vi "FlatToRichnixnet_grpc_GetPropertyResponse.vi"(5 "OutputClusterType":T1, 11 "InputCluster":T2) -> (3 "OutputCluster":T1)   [LabVIEW 2025, in "grpc-xnet_client.lvlib"]
uses:
  grpc-xnet_client.lvlib
  nixnet_grpc_GetPropertyResponse_Flat.ctl
  nixnet_grpc_U32Array_Flat.ctl
  nidevice_grpc_Session_Flat.ctl
  nixnet_grpc_DbRefArray_Flat.ctl
  nixnet_grpc_DeviceRefArray_Flat.ctl
  nixnet_grpc_InterfaceRefArray_Flat.ctl
  nixnet_grpc_EptRxFilterArray_Flat.ctl
  nixnet_grpc_EptRxFilter_Flat.ctl
  nixnet_grpc_GetPropertyResponse.ctl
  nixnet_grpc_GetPropertyResponse_property_value/nixnet_grpc_GetPropertyResponse_property_value.lvclass
  nixnet_grpc_GetPropertyResponse_property_value/nixnet_grpc_GetPropertyResponse_property_value.lvclass/nixnet_grpc_GetPropertyResponse_property_value.ctl
  FlatToRichnixnet_grpc_EptRxFilter.vi
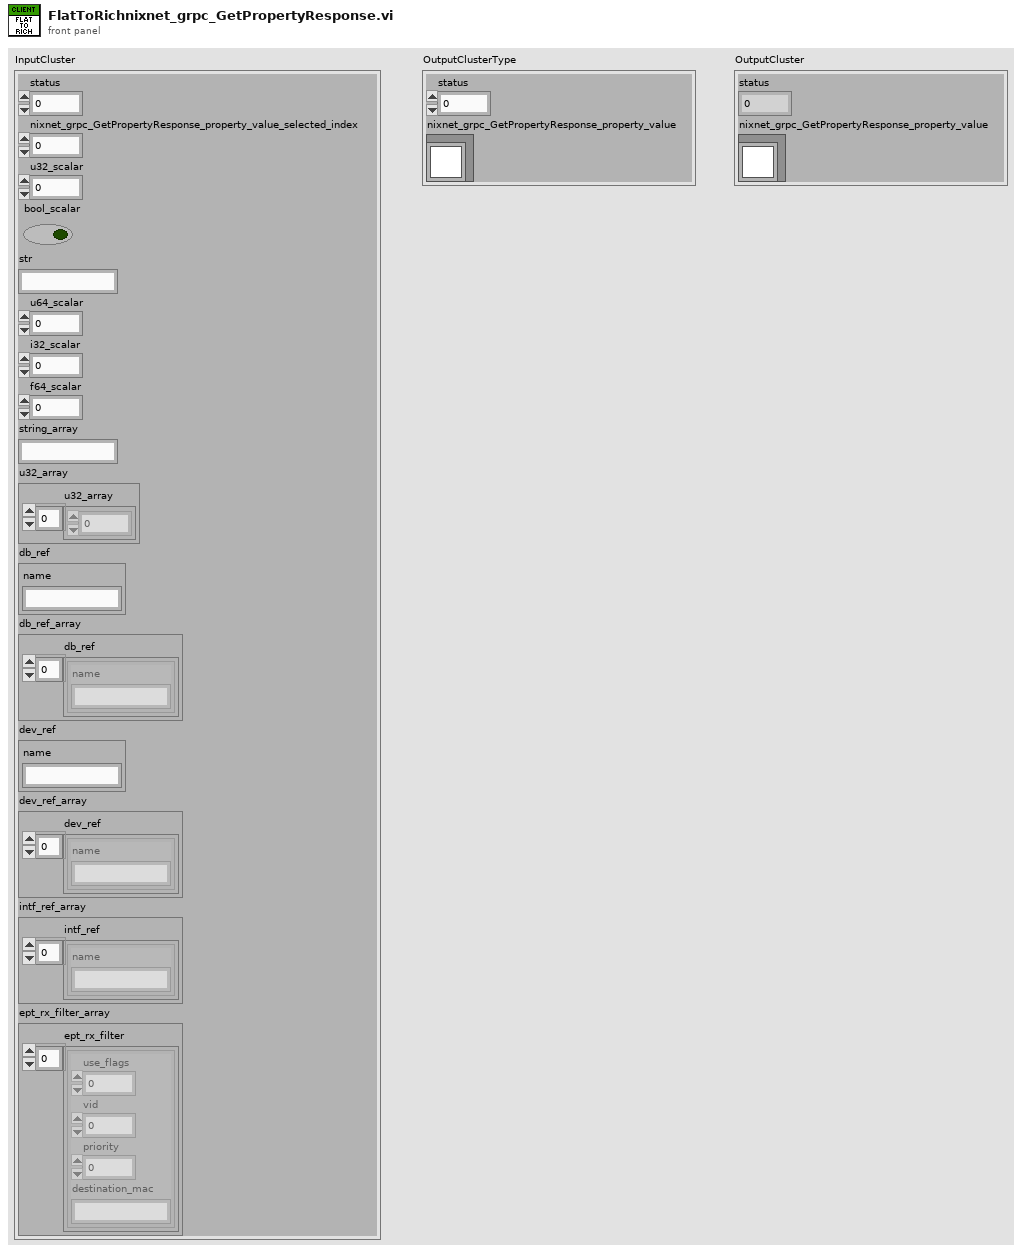
[diagram p1: front panel]
types:
  T1 = typedef "grpc-xnet_client.lvlib/nixnet_grpc_GetPropertyResponse.ctl" = cluster{"status":i32, "nixnet_grpc_GetPropertyResponse_property_value":refnum<class "nixnet_grpc_GetPropertyResponse_property_value.lvclass">}
  T2 = typedef "grpc-xnet_client.lvlib/nixnet_grpc_GetPropertyResponse_Flat.ctl" = cluster{"status":i32, "nixnet_grpc_GetPropertyResponse_property_value_selected_index":i32, "u32_scalar":u32, "bool_scalar":bool, "str":string, "u64_scalar":u64, "i32_scalar":i32, "f64_scalar":dbl, "string_array":string, "u32_array":T3, "db_ref":T4, "db_ref_array":T5, "dev_ref":T4, "dev_ref_array":T6, "intf_ref_array":T7, "ept_rx_filter_array":T8}
  T3 = typedef "grpc-xnet_client.lvlib/nixnet_grpc_U32Array_Flat.ctl" = cluster{"u32_array":u32[]}
  T4 = typedef "grpc-xnet_client.lvlib/nidevice_grpc_Session_Flat.ctl" = cluster{"name":string}
  T5 = typedef "grpc-xnet_client.lvlib/nixnet_grpc_DbRefArray_Flat.ctl" = cluster{"db_ref":T4[]}
  T6 = typedef "grpc-xnet_client.lvlib/nixnet_grpc_DeviceRefArray_Flat.ctl" = cluster{"dev_ref":T4[]}
  T7 = typedef "grpc-xnet_client.lvlib/nixnet_grpc_InterfaceRefArray_Flat.ctl" = cluster{"intf_ref":T4[]}
  T8 = typedef "grpc-xnet_client.lvlib/nixnet_grpc_EptRxFilterArray_Flat.ctl" = cluster{"ept_rx_filter":T9[]}
  T9 = typedef "grpc-xnet_client.lvlib/nixnet_grpc_EptRxFilter_Flat.ctl" = cluster{"use_flags":u32, "vid":u32, "priority":u32, "destination_mac":string}
  T10 = typedef "grpc-xnet_client.lvlib/nixnet_grpc_U32Array.ctl" = cluster{"u32_array":u32[]}
  T11 = typedef "grpc-xnet_client.lvlib/nidevice_grpc_Session.ctl" = cluster{"name":string}
  T12 = typedef "grpc-xnet_client.lvlib/nixnet_grpc_DbRefArray.ctl" = cluster{"db_ref":T11[]}
  T13 = typedef "grpc-xnet_client.lvlib/nixnet_grpc_DeviceRefArray.ctl" = cluster{"dev_ref":T11[]}
  T14 = typedef "grpc-xnet_client.lvlib/nixnet_grpc_InterfaceRefArray.ctl" = cluster{"intf_ref":T11[]}
  T15 = typedef "grpc-xnet_client.lvlib/nixnet_grpc_EptRxFilterArray.ctl" = cluster{"ept_rx_filter":T16[]}
  T16 = typedef "grpc-xnet_client.lvlib/nixnet_grpc_EptRxFilter.ctl" = cluster{"use_flags":u32, "vid":u32, "priority":u32, "destination_mac":string}
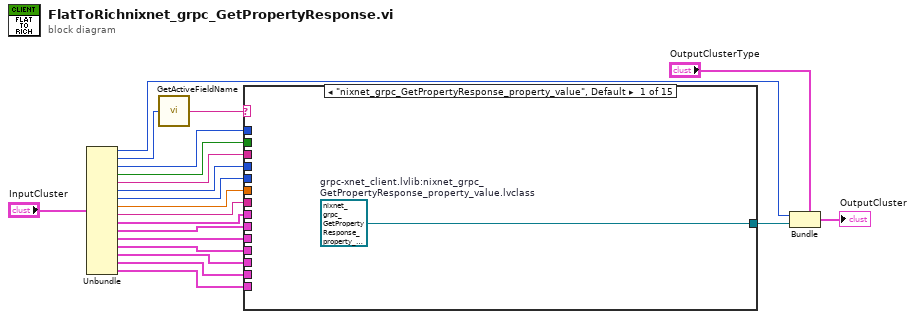
[diagram p0: block diagram]
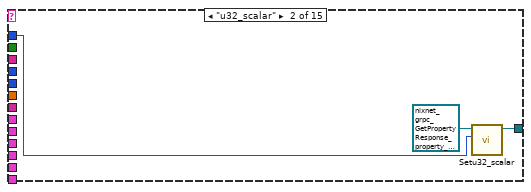
[diagram p2: hidden frame]
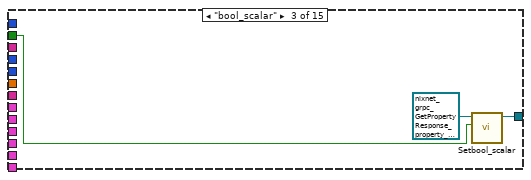
[diagram p3: hidden frame]
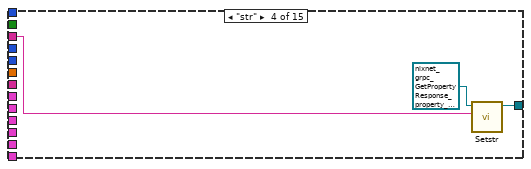
[diagram p4: hidden frame]
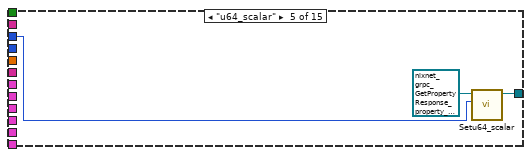
[diagram p5: hidden frame]
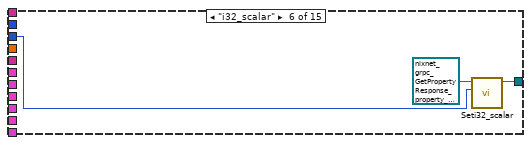
[diagram p6: hidden frame]
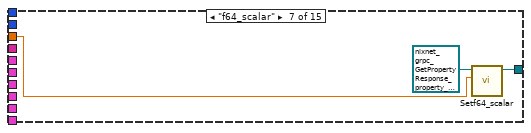
[diagram p7: hidden frame]
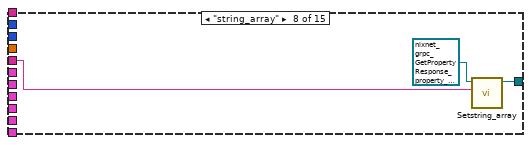
[diagram p8: hidden frame]
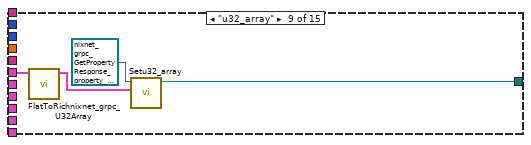
[diagram p9: hidden frame]
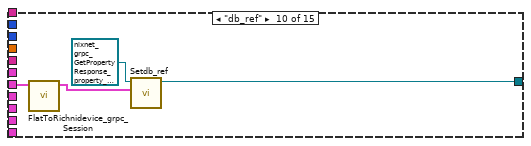
[diagram p10: hidden frame]
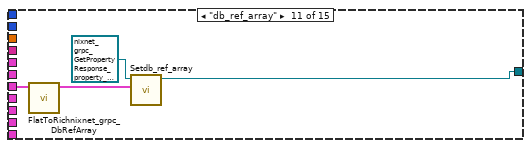
[diagram p11: hidden frame]
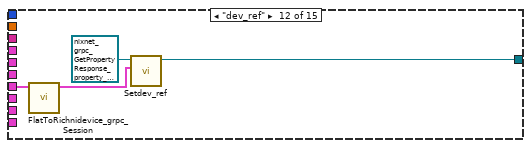
[diagram p12: hidden frame]
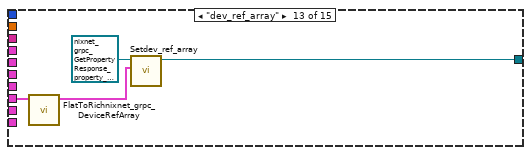
[diagram p13: hidden frame]
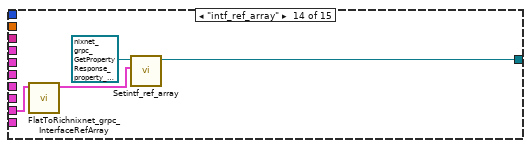
[diagram p14: hidden frame]
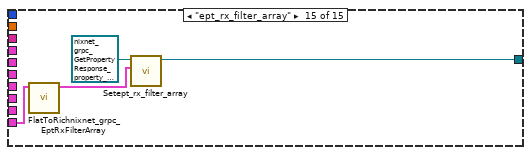
[diagram p15: hidden frame]
diagram:
  n1 = Unbundle "Unbundle"("InputCluster") -> ("status"=w18:i32, "nixnet_grpc_GetPropertyResponse_property_value_selected_index"=w17:i32, "u32_scalar"=w14:u32, "bool_scalar"=w13:bool, "str"=w12:string, "u64_scalar"=w11:u64, "i32_scalar"=w10:i32, "f64_scalar"=w9:dbl, "string_array"=w8:string, "u32_array"=w7:T3, "db_ref"=w6:T4, "db_ref_array"=w5:T5, "dev_ref"=w4:T4, "dev_ref_array"=w3:T6, "intf_ref_array"=w2:T7, "ept_rx_filter_array"=w1:T8)
  n2 = call "GetActiveFieldName.vi"("protobuf index"=w17) -> ("oneof field name"=w16:string)
  n3 = case "nixnet_grpc_GetPropertyResponse_property_value" shown="\"nixnet_grpc_GetPropertyResponse_property_value\", Default" w16 {
    tunnel: [w22 w24 w27 w30 w33 w36 w39 w42 w45 w49 w53 w57 w61 w65 w69] -> w15
    tunnel: w14 -> [_ w25 _ _ _ _ _ _ _ _ _ _ _ _ _]
    tunnel: w13 -> [_ _ w28 _ _ _ _ _ _ _ _ _ _ _ _]
    tunnel: w12 -> [_ _ _ w31 _ _ _ _ _ _ _ _ _ _ _]
    tunnel: w11 -> [_ _ _ _ w34 _ _ _ _ _ _ _ _ _ _]
    tunnel: w10 -> [_ _ _ _ _ w37 _ _ _ _ _ _ _ _ _]
    tunnel: w9 -> [_ _ _ _ _ _ w40 _ _ _ _ _ _ _ _]
    tunnel: w8 -> [_ _ _ _ _ _ _ w43 _ _ _ _ _ _ _]
    tunnel: w7 -> [_ _ _ _ _ _ _ _ w47 _ _ _ _ _ _]
    tunnel: w6 -> [_ _ _ _ _ _ _ _ _ w51 _ _ _ _ _]
    tunnel: w5 -> [_ _ _ _ _ _ _ _ _ _ w55 _ _ _ _]
    tunnel: w4 -> [_ _ _ _ _ _ _ _ _ _ _ w59 _ _ _]
    tunnel: w3 -> [_ _ _ _ _ _ _ _ _ _ _ _ w63 _ _]
    tunnel: w2 -> [_ _ _ _ _ _ _ _ _ _ _ _ _ w67 _]
    tunnel: w1 -> [_ _ _ _ _ _ _ _ _ _ _ _ _ _ w71]
    frame "nixnet_grpc_GetPropertyResponse_property_value", Default {
      w22 = refnum<class "nixnet_grpc_GetPropertyResponse_property_value.lvclass"> refnum  # grpc-xnet_client.lvlib:nixnet_grpc_GetPropertyResponse_property_value.lvclass
    }
    frame "u32_scalar" {
      n4 = call "Setu32_scalar.vi"("Set_Val"=w25, "OneOfTemplate in"=refnum<class "nixnet_grpc_GetPropertyResponse_property_value.lvclass"> refnum) -> ("OneOfTemplate out"=w24:refnum<class "nixnet_grpc_GetPropertyResponse_property_value.lvclass">)  [unwired: 8 in, 1 out]
    }
    frame "bool_scalar" {
      n5 = call "Setbool_scalar.vi"("Set_Val"=w28, "OneOfTemplate in"=refnum<class "nixnet_grpc_GetPropertyResponse_property_value.lvclass"> refnum) -> ("OneOfTemplate out"=w27:refnum<class "nixnet_grpc_GetPropertyResponse_property_value.lvclass">)  [unwired: 8 in, 1 out]
    }
    frame "str" {
      n6 = call "Setstr.vi"("Set_Val"=w31, "OneOfTemplate in"=refnum<class "nixnet_grpc_GetPropertyResponse_property_value.lvclass"> refnum) -> ("OneOfTemplate out"=w30:refnum<class "nixnet_grpc_GetPropertyResponse_property_value.lvclass">)  [unwired: 8 in, 1 out]
    }
    frame "u64_scalar" {
      n7 = call "Setu64_scalar.vi"("Set_Val"=w34, "OneOfTemplate in"=refnum<class "nixnet_grpc_GetPropertyResponse_property_value.lvclass"> refnum) -> ("OneOfTemplate out"=w33:refnum<class "nixnet_grpc_GetPropertyResponse_property_value.lvclass">)  [unwired: 8 in, 1 out]
    }
    frame "i32_scalar" {
      n8 = call "Seti32_scalar.vi"("Set_Val"=w37, "OneOfTemplate in"=refnum<class "nixnet_grpc_GetPropertyResponse_property_value.lvclass"> refnum) -> ("OneOfTemplate out"=w36:refnum<class "nixnet_grpc_GetPropertyResponse_property_value.lvclass">)  [unwired: 8 in, 1 out]
    }
    frame "f64_scalar" {
      n9 = call "Setf64_scalar.vi"("Set_Val"=w40, "OneOfTemplate in"=refnum<class "nixnet_grpc_GetPropertyResponse_property_value.lvclass"> refnum) -> ("OneOfTemplate out"=w39:refnum<class "nixnet_grpc_GetPropertyResponse_property_value.lvclass">)  [unwired: 8 in, 1 out]
    }
    frame "string_array" {
      n10 = call "Setstring_array.vi"("Set_Val"=w43, "OneOfTemplate in"=refnum<class "nixnet_grpc_GetPropertyResponse_property_value.lvclass"> refnum) -> ("OneOfTemplate out"=w42:refnum<class "nixnet_grpc_GetPropertyResponse_property_value.lvclass">)  [unwired: 8 in, 1 out]
    }
    frame "u32_array" {
      n11 = call "FlatToRichnixnet_grpc_U32Array.vi"("InputCluster"=w47) -> ("OutputCluster"=w46:T10)  [unwired: 10 in]
      n12 = call "Setu32_array.vi"("Set_Val"=w46, "OneOfTemplate in"=refnum<class "nixnet_grpc_GetPropertyResponse_property_value.lvclass"> refnum) -> ("OneOfTemplate out"=w45:refnum<class "nixnet_grpc_GetPropertyResponse_property_value.lvclass">)  [unwired: 8 in, 1 out]
    }
    frame "db_ref" {
      n13 = call "FlatToRichnidevice_grpc_Session.vi"("InputCluster"=w51) -> ("OutputCluster"=w50:T11)  [unwired: 10 in]
      n14 = call "Setdb_ref.vi"("Set_Val"=w50, "OneOfTemplate in"=refnum<class "nixnet_grpc_GetPropertyResponse_property_value.lvclass"> refnum) -> ("OneOfTemplate out"=w49:refnum<class "nixnet_grpc_GetPropertyResponse_property_value.lvclass">)  [unwired: 8 in, 1 out]
    }
    frame "db_ref_array" {
      n15 = call "FlatToRichnixnet_grpc_DbRefArray.vi"("InputCluster"=w55) -> ("OutputCluster"=w54:T12)  [unwired: 10 in]
      n16 = call "Setdb_ref_array.vi"("Set_Val"=w54, "OneOfTemplate in"=refnum<class "nixnet_grpc_GetPropertyResponse_property_value.lvclass"> refnum) -> ("OneOfTemplate out"=w53:refnum<class "nixnet_grpc_GetPropertyResponse_property_value.lvclass">)  [unwired: 8 in, 1 out]
    }
    frame "dev_ref" {
      n17 = call "FlatToRichnidevice_grpc_Session.vi"("InputCluster"=w59) -> ("OutputCluster"=w58:T11)  [unwired: 10 in]
      n18 = call "Setdev_ref.vi"("Set_Val"=w58, "OneOfTemplate in"=refnum<class "nixnet_grpc_GetPropertyResponse_property_value.lvclass"> refnum) -> ("OneOfTemplate out"=w57:refnum<class "nixnet_grpc_GetPropertyResponse_property_value.lvclass">)  [unwired: 8 in, 1 out]
    }
    frame "dev_ref_array" {
      n19 = call "FlatToRichnixnet_grpc_DeviceRefArray.vi"("InputCluster"=w63) -> ("OutputCluster"=w62:T13)  [unwired: 10 in]
      n20 = call "Setdev_ref_array.vi"("Set_Val"=w62, "OneOfTemplate in"=refnum<class "nixnet_grpc_GetPropertyResponse_property_value.lvclass"> refnum) -> ("OneOfTemplate out"=w61:refnum<class "nixnet_grpc_GetPropertyResponse_property_value.lvclass">)  [unwired: 8 in, 1 out]
    }
    frame "intf_ref_array" {
      n21 = call "FlatToRichnixnet_grpc_InterfaceRefArray.vi"("InputCluster"=w67) -> ("OutputCluster"=w66:T14)  [unwired: 10 in]
      n22 = call "Setintf_ref_array.vi"("Set_Val"=w66, "OneOfTemplate in"=refnum<class "nixnet_grpc_GetPropertyResponse_property_value.lvclass"> refnum) -> ("OneOfTemplate out"=w65:refnum<class "nixnet_grpc_GetPropertyResponse_property_value.lvclass">)  [unwired: 8 in, 1 out]
    }
    frame "ept_rx_filter_array" {
      n23 = call "FlatToRichnixnet_grpc_EptRxFilterArray.vi"("InputCluster"=w71) -> ("OutputCluster"=w70:T15)  [unwired: 10 in]
      n24 = call "Setept_rx_filter_array.vi"("Set_Val"=w70, "OneOfTemplate in"=refnum<class "nixnet_grpc_GetPropertyResponse_property_value.lvclass"> refnum) -> ("OneOfTemplate out"=w69:refnum<class "nixnet_grpc_GetPropertyResponse_property_value.lvclass">)  [unwired: 8 in, 1 out]
    }
  }
  n25 = Bundle "Bundle"(cluster="OutputClusterType", "status"=w18, "nixnet_grpc_GetPropertyResponse_property_value"=w15) -> (→"OutputCluster":T1)
